vi "Introspection Core.vi"(8 "error in (no error)":errorcluster, 11 "CS++DeviceActor in":refnum<class "CS++DeviceActor.lvclass">) -> (0 "error out":errorcluster, 2 "CS++Messages":refnum<class "Message.lvclass">[](array[class]), 3 "CS++DeviceActor out":refnum<class "CS++DeviceActor.lvclass">)   [LabVIEW 2016, in "CS++DeviceActor.lvlib" / "CS++DeviceActor.lvclass"]
doc: "This vi delivers a list with all messages this actor reacts to. \n\nNote that all inherited classes have to overwrite it."
uses:
  CS++DeviceActor.lvclass
  <vilib>/ActorFramework/Message/Message.lvclass
  CS++DeviceActor Messages/Reset Device Msg/Reset Device Msg.lvclass
  C:/Program Files (x86)/National Instruments/LabVIEW 2016/vi.lib/ActorFramework/Message/Message.lvclass
  CS++DeviceActor Messages/Selftest Device Msg/Selftest Device Msg.lvclass
  CS++BaseActor/CS++BaseActor.lvclass
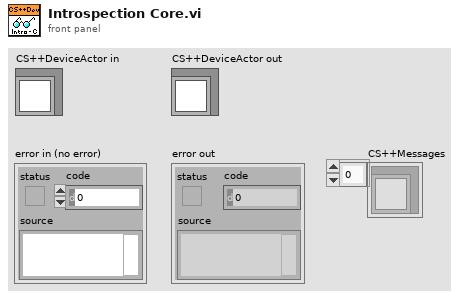
[diagram p1: front panel]
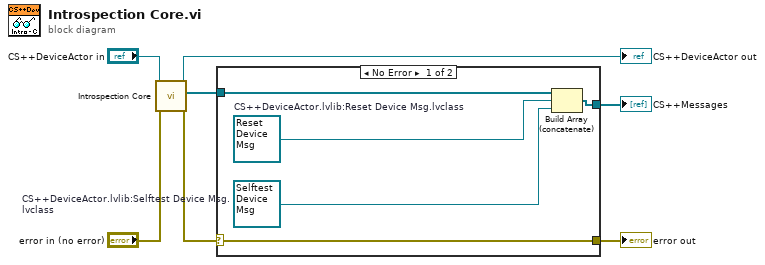
[diagram p0: block diagram]
diagram:
  n1 = call-parent "Introspection Core.vi"("error in (no error)"="error in (no error)", "CS++BaseActor in"="CS++DeviceActor in") -> ("error out"=w4:errorcluster, "CS++Messages"=w2:refnum<class "Message.lvclass">[], "CS++BaseActor out"=→"CS++DeviceActor out":refnum<class "CS++DeviceActor.lvclass">)  [unwired: 7 in]
  n2 = case shown="No Error" w4 {
    selector: w4 -> [w12 w13]
    tunnel: [w12 w13] -> w3
    tunnel: w2 -> [w11 _]
    tunnel: [w8 _] -> w1
    frame No Error {
      w9 = refnum<class "Selftest Device Msg.lvclass"> refnum  # CS++DeviceActor.lvlib:Selftest Device Msg.lvclass
      w10 = refnum<class "Reset Device Msg.lvclass"> refnum  # CS++DeviceActor.lvlib:Reset Device Msg.lvclass
      n3 = Build Array (concatenate)(w11, w10, w9) -> (w8:refnum<class "Message.lvclass">[])
    }
    frame Error {
    }
  }
  "error out" <- w3
  "CS++Messages" <- w1
